vi "Brent with Derivatives 1D_core(VI).vi"(4 "sign":i32(ring) items=["y=f(x)", "y=-f(x)"], 5 "accuracy":dbl=1e-08 format="%.0e", 6 "data":variant, 7 "f(x)":T1, 8 "error in":i32, 9 "c (start)":dbl format="%.2f", 10 "b (start)":dbl format="%.2f", 11 "a (start)":dbl format="%.2f") -> (0 "error out":i32, 1 "ticks":u32, 2 "f(minimum)":dbl format="%.2f", 3 "minimum":dbl format="%.2f")   [LabVIEW 2020, in "NI_Gmath.lvlib"]
uses:
  <vilib>/gmath/NI_Gmath.lvlib
  <vilib>/gmath/_ref_NR.llb/functionRefnum.ctl
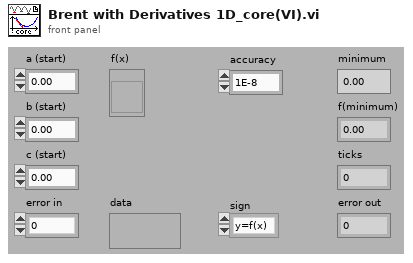
[diagram p1: front panel]
types:
  T1 = typedef "NI_Gmath.lvlib/functionRefnum.ctl" = refnum<vi>
  T2 = cluster{"c (start)":dbl, "c (start)":dbl, "c (start)":dbl}
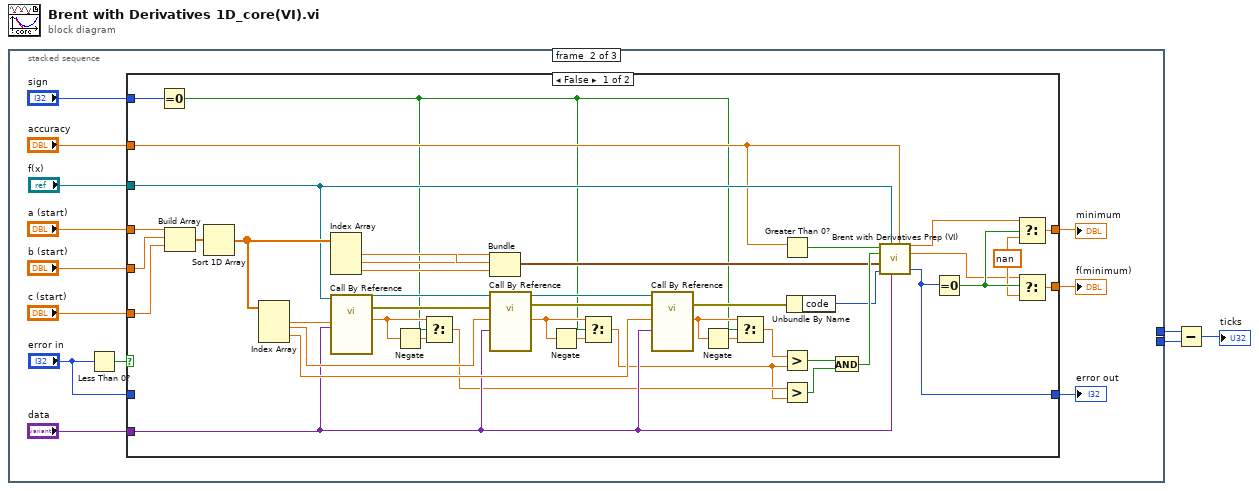
[diagram p0: block diagram]
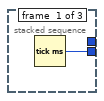
[diagram p2: hidden frame]
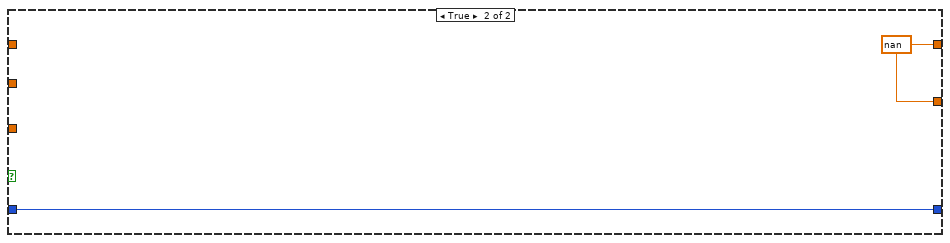
[diagram p3: hidden frame]
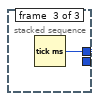
[diagram p4: hidden frame]
diagram:
  n1 = stacked-sequence {
    tunnel: [w4 _ _] -> w2
    tunnel: [_ _ w62] -> w1
    frame #0 {
      n2 = Tick Count (ms)() -> (millisecond timer value=w4:u32)
    }
    frame #1 {
      n3 = Less Than 0?(x="error in") -> (x < 0?=w13:bool)
      n4 = case shown="False" w13 {
        tunnel: [w56 w61] -> w16
        tunnel: [w54 w61] -> w15
        tunnel: [w47 w60] -> w14
        tunnel: "error in" -> [_ w60]
        tunnel: "f(x)" -> [w36 _]
        tunnel: "accuracy" -> [w32 _]
        tunnel: "a (start)" -> [w31 _]
        tunnel: "b (start)" -> [w30 _]
        tunnel: "c (start)" -> [w29 _]
        tunnel: "data" -> [w28 _]
        tunnel: "sign" -> [w26 _]
        frame False {
          w53 = nan
          n5 = Equal To 0?(x=w26) -> (x = 0?=w17:bool)
          n6 = Build Array(w31, w30, w29) -> (w58:dbl[])
          n7 = Sort 1D Array(array=w58) -> (sorted array=w42:dbl[])
          n8 = Index Array(array=w42) -> (element #1=w41:dbl, element #2=w40:dbl, element #3=w39:dbl)  [unwired: 3 in]
          n9 = Index Array(array=w42) -> (element #1=w51:dbl, element #2=w50:dbl, element #3=w49:dbl)  [unwired: 3 in]
          n10 = call-by-ref "?"(reference=w36, "Variant"=w28, "x"=w41) -> (reference out=w44:T1, error out=w35:errorcluster, 2:"f(x)"=w25:dbl)  [unwired: 4 in]
          n11 = Negate(x=w25) -> (-x=w27:dbl)
          n12 = Select(t=w25, s=w17, f=w27) -> (s? t:f=w24:dbl)
          n13 = Bundle("c (start)"=w50, "c (start)"=w51, "c (start)"=w49) -> (w48:T2)  [unwired: 1 out]
          n14 = call-by-ref "?"(reference=w44, error in=w35, "Variant"=w28, "x"=w40) -> (reference out=w43:T1, error out=w34:errorcluster, 2:"f(x)"=w22:dbl)  [unwired: 3 in]
          n15 = Negate(x=w22) -> (-x=w23:dbl)
          n16 = Select(t=w22, s=w17, f=w23) -> (s? t:f=w21:dbl)
          n17 = call-by-ref "?"(reference=w43, error in=w34, "Variant"=w28, "x"=w39) -> (error out=w33:errorcluster, "f(x)"=w18:dbl)  [unwired: 3 in, 1 out]
          n18 = Negate(x=w18) -> (-x=w20:dbl)
          n19 = Select(t=w18, s=w17, f=w20) -> (s? t:f=w19:dbl)
          n20 = Greater Than 0?(x=w32) -> (x > 0?=w38:bool)
          n21 = Greater?(x=w19, y=w21) -> (0:w59:bool)
          n22 = Greater?(x=w24, y=w21) -> (0:w57:bool)
          n23 = Unbundle By Name(w33) -> ("code"=w37:i32)
          n24 = And(x=w59, y=w57) -> (x .and. y?=w52:bool)
          n25 = call <vilib>:"Brent with Derivatives Prep (VI).vi"("accuracy"=w32, "data"=w28, "f(x)"=w36, "error in"=w37, "values"=w48, "inner case"=w52, "outer case"=w38) -> ("error out"=w47:i32, "f(minimum)"=w46:dbl, "minimum"=w45:dbl)  [unwired: 1 in, 1 out]
          n26 = Equal To 0?(x=w47) -> (x = 0?=w55:bool)
          n27 = Select(t=w45, s=w55, f=w53) -> (s? t:f=w54:dbl)
          n28 = Select(t=w46, s=w55, f=w53) -> (s? t:f=w56:dbl)
        }
        frame True {
          w61 = nan ("minimum")
        }
      }
      "f(minimum)" <- w16
      "minimum" <- w15
      "error out" <- w14
    }
    frame #2 {
      n29 = Tick Count (ms)() -> (millisecond timer value=w62:u32)
    }
  }
  n30 = Subtract(x=w1, y=w2) -> (x-y=→"ticks":u32)
